vi "GFITS_LibGetMemFits.vi"(8 "error in (no error)":errorcluster) -> (0 "error out":errorcluster, 2 "memfits":bool)   [LabVIEW 2016]
uses:
  c/lib/libgfits.so
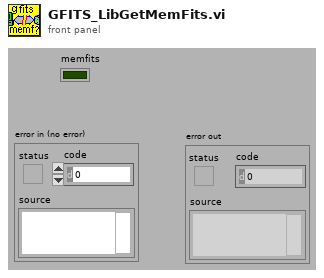
[diagram p1: front panel]
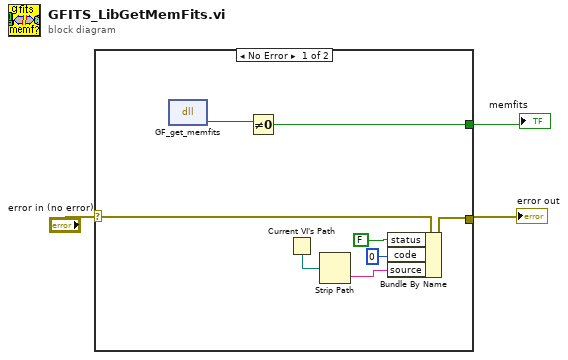
[diagram p0: block diagram]
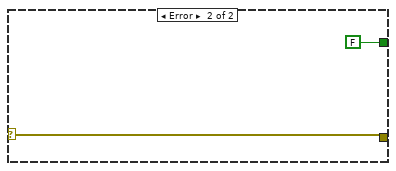
[diagram p2: hidden frame]
diagram:
  n1 = case shown="No Error" "error in (no error)" {
    selector: "error in (no error)" -> [w11 w13]
    tunnel: [w8 w13] -> w2
    tunnel: [w4 FALSE] -> w1
    frame No Error {
      n2 = dll-call lib="home/simager/panview/PAN/Modules/GFITS/private/c/lib/libgfits.so" fn="GF_get_memfits"() -> ("return type"=w5:i16)  [unwired: 3 in, 2 out]
      n3 = Not Equal To 0?(x=w5) -> (x != 0?=w4:bool)
      n4 = Current VI's Path() -> (path=w10:path)
      n5 = Strip Path(path=w10) -> (name=w9:string)  [unwired: 1 out]
      n6 = Bundle By Name(cluster=w11, "status"=FALSE, "code"=0, "source"=w9) -> (w8:errorcluster)
    }
    frame Error {
    }
  }
  "error out" <- w2
  "memfits" <- w1
